vi "ROI_Image_Determine Intersection of line and circle.vi"(8 "error in (no error)":errorcluster, 10 "Circles Data":T2, 11 "Start Point":cluster{"X":i32, "Y":i32}) -> (0 "error out":errorcluster, 1 "Orient rel to center":T1, 2 "Intersection point":cluster{"X":i32, "Y":i32})   [LabVIEW 2014]
uses:
  custom controls/enum - StartPt Relative to Circle Center.ctl
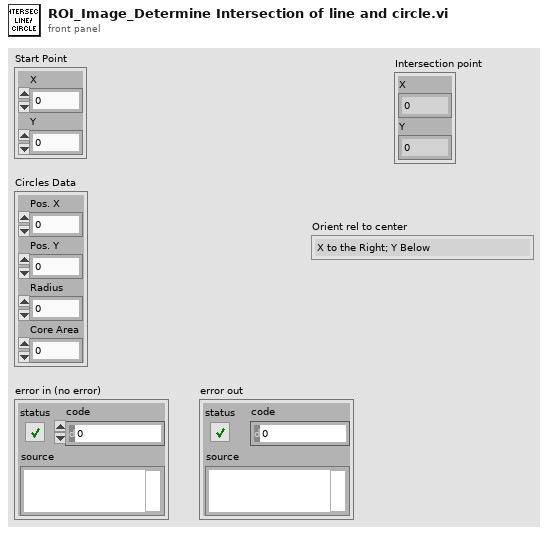
[diagram p1: front panel]
types:
  T1 = typedef "enum - StartPt Relative to Circle Center.ctl" = enum16{"X to the Right; Y Below", "X to the Right; Y Above", "X to the Left; Y Below", "X to the Left: Y Above"}
  T2 = cluster{"Pos. X":i32, "Pos. Y":i32, "Radius":i32, "Core Area":i32}
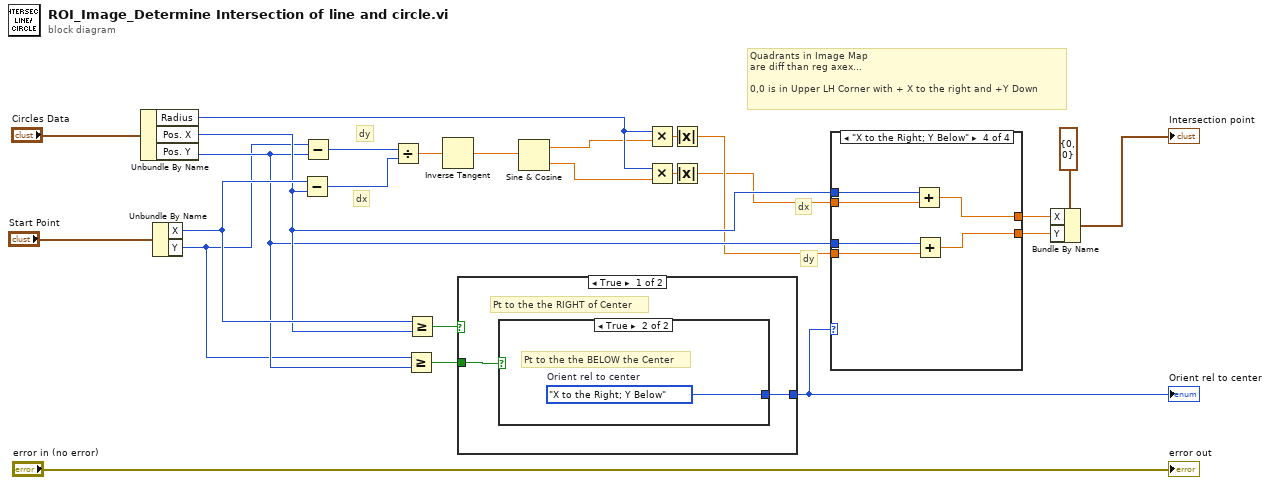
[diagram p0: block diagram]
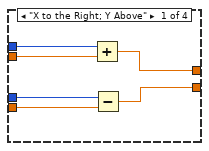
[diagram p2: hidden frame]
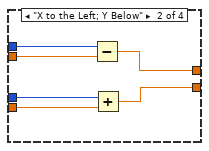
[diagram p3: hidden frame]
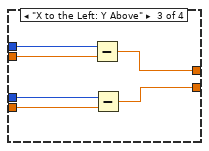
[diagram p4: hidden frame]
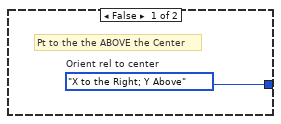
[diagram p5: hidden frame]
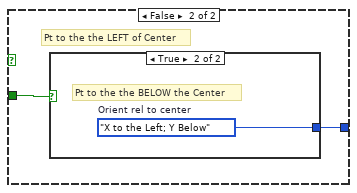
[diagram p6: hidden frame]
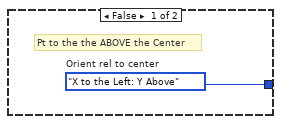
[diagram p7: hidden frame]
diagram:
  # "dx"
  # "dy"
  # "Quadrants in Image Map\nare diff than reg axex...\n\n0,0 is in Upper LH Corner with + X to the right and +Y Down"
  # "dx"
  # "dy"
  n1 = Unbundle By Name("Circles Data") -> ("Radius"=w22:i32, "Pos. X"=w10:i32, "Pos. Y"=w9:i32)
  n2 = Unbundle By Name("Start Point") -> ("X"=w11:i32, "Y"=w8:i32)
  n3 = Subtract(x=w11, y=w10) -> (x-y=w3:i32)
  n4 = Subtract(x=w8, y=w9) -> (x-y=w4:i32)
  n5 = Divide(x=w4, y=w3) -> (x/y=w13:dbl)
  n6 = Greater Or Equal?(x=w8, y=w9) -> (x >= y?=w6:bool)
  n7 = Greater Or Equal?(x=w11, y=w10) -> (x >= y?=w7:bool)
  n8 = Inverse Tangent(1:w13) -> (0:w12:dbl)
  n9 = case shown="True" w7 {
    tunnel: w6 -> [w27 w31]
    tunnel: [w26 w30] -> w5
    frame True {
      # "Pt to the the RIGHT of Center"
      n10 = case shown="True" w27 {
        tunnel: [w28 w29] -> w26
        frame False {
          w28 = enum_-_StartPt_Relative_to_Circle_Center."X to the Right; Y Above"  # Orient rel to center
          # "Pt to the the ABOVE the Center"
        }
        frame True {
          w29 = enum_-_StartPt_Relative_to_Circle_Center."X to the Right; Y Below"  # Orient rel to center
          # "Pt to the the BELOW the Center"
        }
      }
    }
    frame False {
      # "Pt to the the LEFT of Center"
      n11 = case shown="True" w31 {
        tunnel: [w32 w33] -> w30
        frame False {
          w32 = enum_-_StartPt_Relative_to_Circle_Center."X to the Left: Y Above"  # Orient rel to center
          # "Pt to the the ABOVE the Center"
        }
        frame True {
          w33 = enum_-_StartPt_Relative_to_Circle_Center."X to the Left; Y Below"  # Orient rel to center
          # "Pt to the the BELOW the Center"
        }
      }
    }
  }
  "Orient rel to center" <- w5
  n12 = Sine & Cosine(0:w12) -> (1:w21:dbl, 2:w19:dbl)
  n13 = Multiply(x=w22, y=w21) -> (x*y=w16:dbl)
  n14 = Multiply(x=w22, y=w19) -> (x*y=w18:dbl)
  n15 = Absolute Value(x=w16) -> (abs(x)=w2:dbl)
  n16 = Absolute Value(x=w18) -> (abs(x)=w1:dbl)
  n17 = case shown="\"X to the Right; Y Below\"" w5 {
    tunnel: w1 -> [w39 w45 w51 w57]
    tunnel: [w38 w44 w50 w56] -> w17
    tunnel: w2 -> [w37 w43 w49 w55]
    tunnel: [w36 w42 w48 w54] -> w15
    tunnel: w10 -> [w35 w41 w47 w53]
    tunnel: w9 -> [w34 w40 w46 w52]
    frame "X to the Right; Y Above" {
      n18 = Add(x=w35, y=w39) -> (x+y=w38:dbl)
      n19 = Subtract(x=w34, y=w37) -> (x-y=w36:dbl)
    }
    frame "X to the Left; Y Below" {
      n20 = Subtract(x=w41, y=w45) -> (x-y=w44:dbl)
      n21 = Add(x=w40, y=w43) -> (x+y=w42:dbl)
    }
    frame "X to the Left: Y Above" {
      n22 = Subtract(x=w47, y=w51) -> (x-y=w50:dbl)
      n23 = Subtract(x=w46, y=w49) -> (x-y=w48:dbl)
    }
    frame "X to the Right; Y Below" {
      n24 = Add(x=w53, y=w57) -> (x+y=w56:dbl)
      n25 = Add(x=w52, y=w55) -> (x+y=w54:dbl)
    }
  }
  n26 = Bundle By Name(cluster=cluster{"X":i32, "Y":i32} {"X"=0, "Y"=0} ("Intersection point"), "X"=w17, "Y"=w15) -> (→"Intersection point":cluster{"X":i32, "Y":i32})
  "error out" <- "error in (no error)"
